vi "createScanArrays.vi"() -> ()   [LabVIEW 2013]
panel:
  out "scan array":i32[][](array[numeric])
  in  "samples/pixel":i32=2 min=2
  in  "resolution":i32=1 min=4
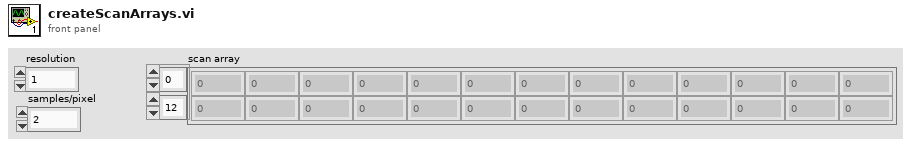
[diagram p1: front panel]
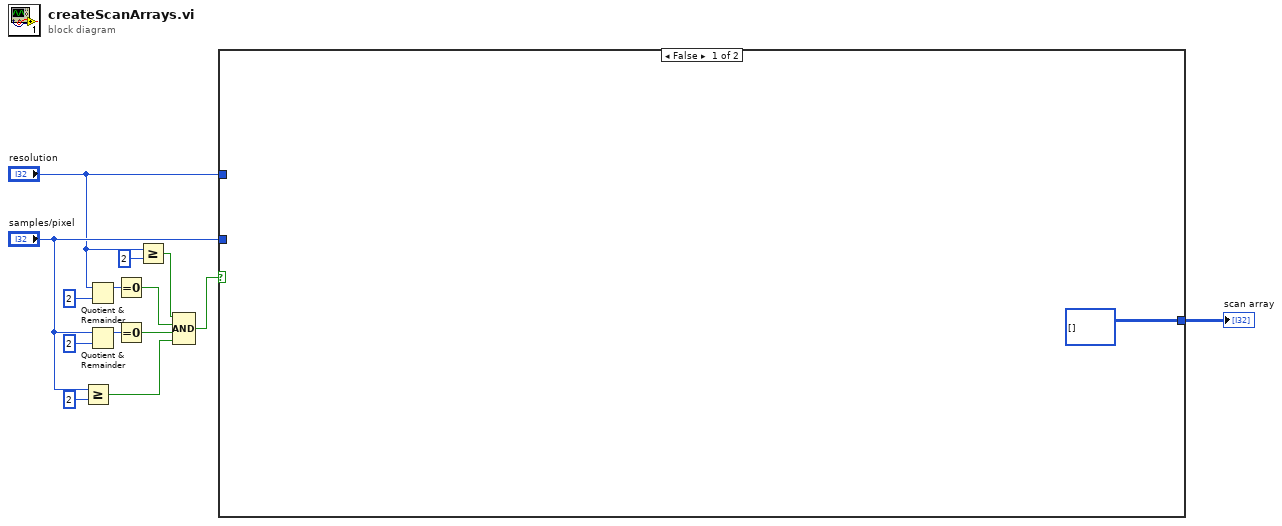
[diagram p0: block diagram]
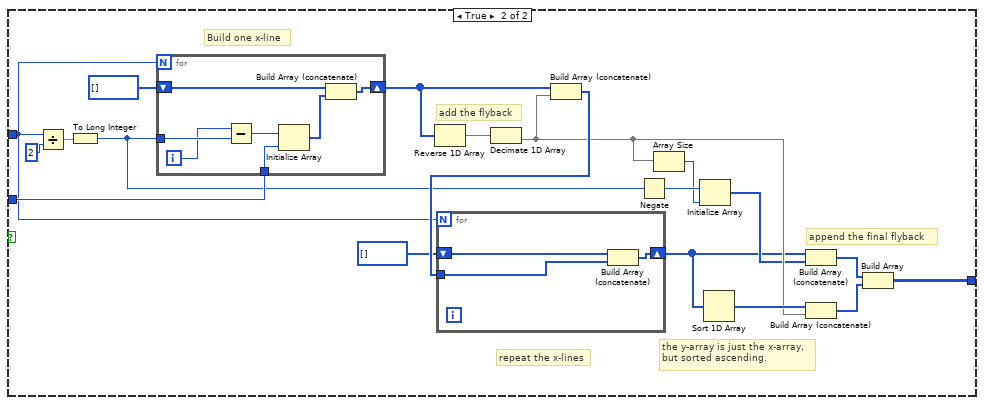
[diagram p2: hidden frame]
diagram:
  n1 = Greater Or Equal?(x="samples/pixel", y=2) -> (x >= y?=w5:bool)
  n2 = Quotient & Remainder(x="resolution", y=2) -> (x-y*floor(x/y)=w13:i32)  [unwired: 1 out]
  n3 = Quotient & Remainder(x="samples/pixel", y=2) -> (x-y*floor(x/y)=w11:i32)  [unwired: 1 out]
  n4 = Equal To 0?(x=w13) -> (x = 0?=w10:bool)
  n5 = Equal To 0?(x=w11) -> (x = 0?=w9:bool)
  n6 = Greater Or Equal?(x="resolution", y=2) -> (x >= y?=w2:bool)
  n7 = Compound Arithmetic op=AND(w2, w10, w9, w5) -> (w8:bool)
  n8 = case shown="False" w8 {
    tunnel: "samples/pixel" -> [_ w30]
    tunnel: "resolution" -> [_ w26]
    tunnel: [i32[][] [] w16] -> w1
    frame False {
    }
    frame True {
      # "add the flyback"
      # "append the final flyback"
      # "the y-array is just the x-array,\nbut sorted ascending."
      # "repeat the x-lines"
      # "Build one x-line"
      n9 = Divide(x=w26, y=2) -> (x/y=w33:dbl)
      n10 = To Long Integer(number=w33) -> (32bit integer=w23:i32)
      n11 = for {
        N: w26 -> [_]
        shift-right: [w39] -> w31
        shift-left: i32[] [] -> [w40]
        tunnel: w23 -> [w44]
        tunnel: w30 -> [w41]
        i -> [w42]
        n12 = Subtract(x=w42, y=w44) -> (x-y=w43:i32)
        n13 = Initialize Array(w43, w41) -> (w38:i32[])
        n14 = Build Array (concatenate)(w40, w38) -> (w39:i32[])
      }
      n15 = Reverse 1D Array(array=w31) -> (reversed array=w32:i32[])
      n16 = Decimate 1D Array(w32) -> (w21:i32[])  [unwired: 1 out]
      n17 = Build Array (concatenate)(w31, w21) -> (w29:i32[])
      n18 = for {
        N: w26 -> [_]
        tunnel: w29 -> [w36]
        shift-right: [w35] -> w19
        shift-left: i32[] [] -> [w37]
        n19 = Build Array (concatenate)(w37, w36) -> (w35:i32[])
      }
      n20 = Negate(x=w23) -> (-x=w24:i32)
      n21 = Array Size(array=w21) -> (size(s)=w22:i32)
      n22 = Initialize Array(w24, w22) -> (w20:i32[])
      n23 = Sort 1D Array(array=w19) -> (sorted array=w25:i32[])
      n24 = Build Array (concatenate)(w19, w20) -> (w18:i32[])
      n25 = Build Array (concatenate)(w25, w21) -> (w17:i32[])
      n26 = Build Array(w18, w17) -> (w16:i32[][])
    }
  }
  "scan array" <- w1
